vi "prueba5_21241028_ElminMejia.vi"() -> ()   [LabVIEW 2012]
panel:
  out "Array":T1(array[cluster]) {"tanque3" scale=0.0..10.0; "tanque2" scale=0.0..10.0; "tanque1" scale=0.0..10.0}
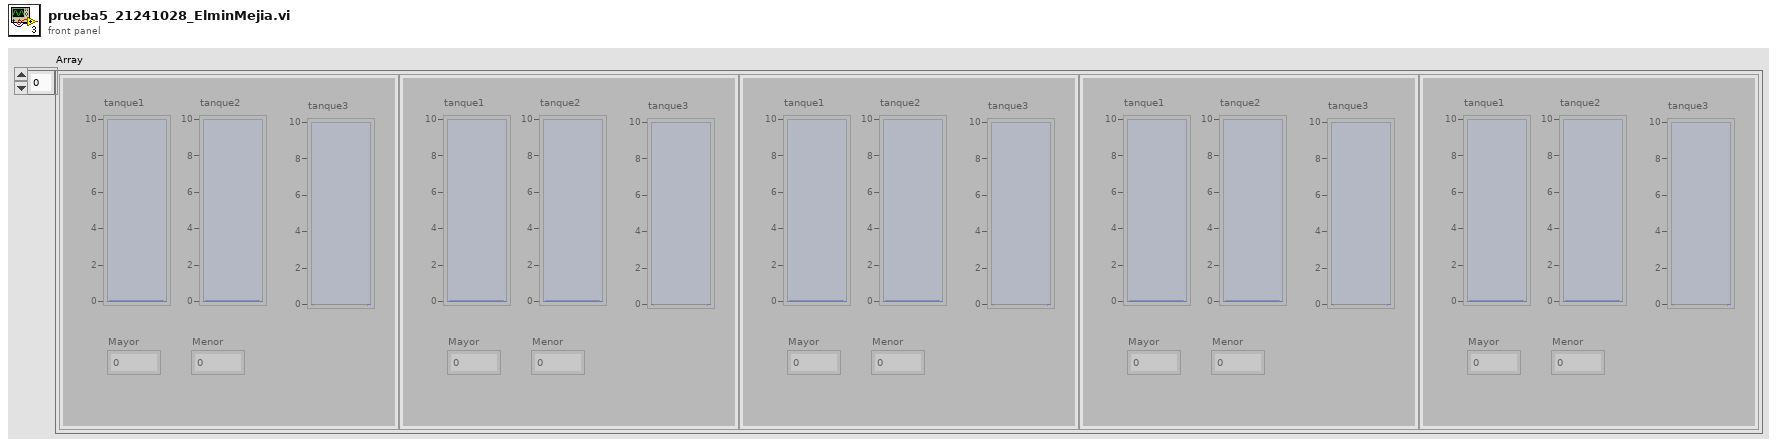
[diagram p1: front panel]
types:
  T1 = cluster{"tanque1":i32, "tanque2":i32, "tanque3":i32, "Mayor":dbl, "Menor":dbl}[]
  T2 = enum16{"open", "replace", "create", "open or create", "replace or create", "replace or create with confirmation"}
  T3 = cluster{"tanque1":i32, "tanque2":i32, "tanque3":i32, "Mayor":dbl, "Menor":dbl}
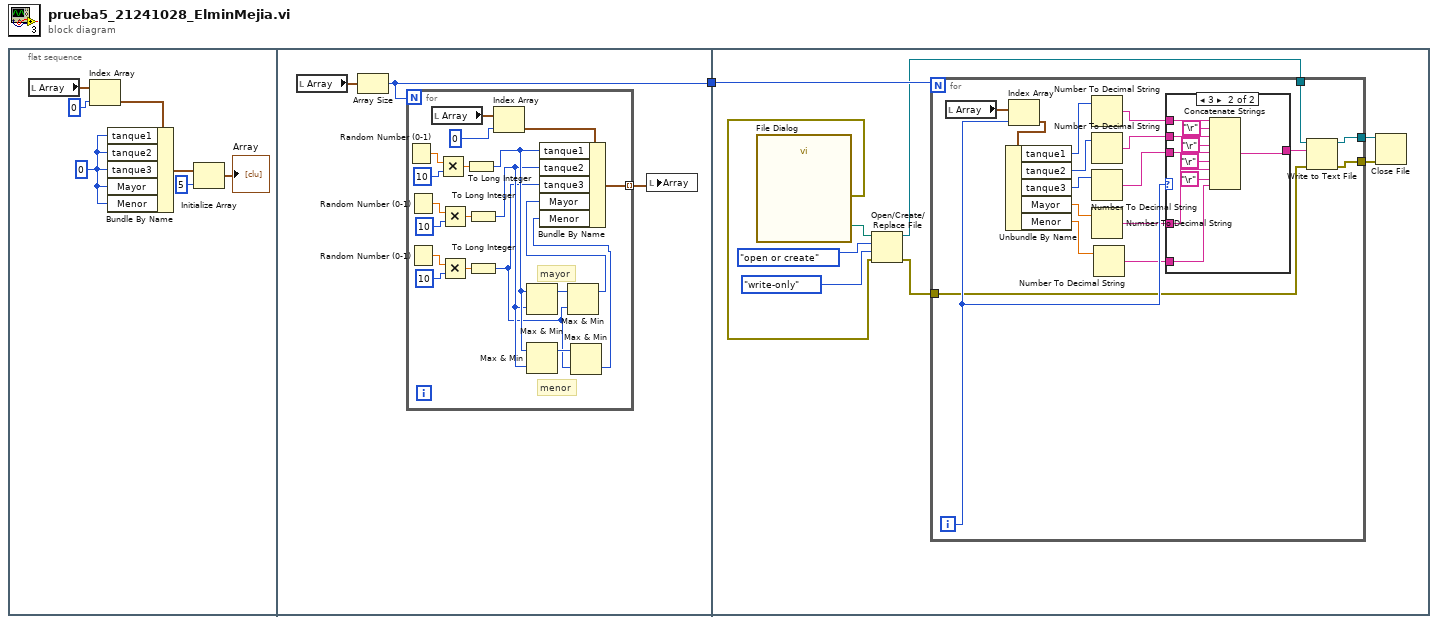
[diagram p0: block diagram]
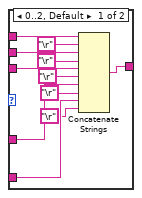
[diagram p2: hidden frame]
diagram:
  n1 = flat-sequence {
    tunnel: [w9] -> w1
    tunnel: w1 -> [w40]
    frame #0 {
      w5 = 0
      n2 = local read "Array"() -> (w8:T1)
      n3 = Index Array(array=w8, index=0) -> (element=w6:T3)
      n4 = Bundle By Name(cluster=w6, "tanque1"=w5, "tanque2"=w5, "tanque3"=w5, "Mayor"=w5, "Menor"=w5) -> (w4:T3)
      n5 = Initialize Array(w4, 5 ("dimension size")) -> (→"Array":T1)
    }
    frame #1 {
      n6 = local read "Array"() -> (w11:T1)
      n7 = Array Size(array=w11) -> (size(s)=w9:i32)
      n8 = for {
        N: w9 -> [_]
        tunnel: [w12] -> w10 mode=indexing
        # "menor"
        # "mayor"
        n9 = Random Number (0-1)() -> (number: 0 to 1=w28:dbl)
        n10 = Random Number (0-1)() -> (number: 0 to 1=w23:dbl)
        n11 = Random Number (0-1)() -> (number: 0 to 1=w22:dbl)
        n12 = local read "Array"() -> (w31:T1)
        n13 = Multiply(x=w28, y=10) -> (x*y=w26:dbl)
        n14 = Multiply(x=w23, y=10) -> (x*y=w25:dbl)
        n15 = Multiply(x=w22, y=10) -> (x*y=w20:dbl)
        n16 = To Long Integer(number=w26) -> (32bit integer=w17:i32)
        n17 = To Long Integer(number=w25) -> (32bit integer=w16:i32)
        n18 = To Long Integer(number=w20) -> (32bit integer=w14:i32)
        n19 = Index Array(array=w31, index=0) -> (element=w29:T3)
        n20 = Max & Min(x=w17, y=w16) -> (max(x,y)=w19:i32)  [unwired: 1 out]
        n21 = Max & Min(x=w17, y=w16) -> (max(x,y)=w15:i32)  [unwired: 1 out]
        n22 = Max & Min(x=w19, y=w14) -> (max(x,y)=w18:i32)  [unwired: 1 out]
        n23 = Max & Min(x=w15, y=w14) -> (min(x,y)=w13:i32)  [unwired: 1 out]
        n24 = Bundle By Name(cluster=w29, "tanque1"=w17, "tanque2"=w16, "tanque3"=w14, "Mayor"=w18, "Menor"=w13) -> (w12:T3)
      }
      n25 = local write "Array"(w10) -> ()
    }
    frame #2 {
      n26 = call "File Dialog"() -> ("selected path"=w39:path, "error out"=w38:errorcluster)  [unwired: 12 in, 2 out]
      n27 = Open/Create/Replace File(file path (use dialog)=w39, error in=w38, operation (0:open)=T2."open or create", access (0:read/write)=enum16{"read/write", "read-only", "write-only"}."write-only") -> (refnum out=w35:refnum<file>, error out=w34:errorcluster)  [unwired: 2 in, 1 out]
      n28 = for {
        N: w40 -> [_]
        tunnel: w35 -> [w44]
        tunnel: w34 -> [w43]
        tunnel: [w42] -> w33
        tunnel: [w41] -> w32
        i -> [w51]
        n29 = local read "Array"() -> (w58:T1)
        n30 = Index Array(array=w58, index=w51) -> (element=w57:T3)
        n31 = Unbundle By Name(w57) -> ("tanque1"=w56:i32, "tanque2"=w55:i32, "tanque3"=w54:i32, "Mayor"=w53:dbl, "Menor"=w52:dbl)
        n32 = Number To Decimal String(number=w56) -> (decimal integer string=w50:string)  [unwired: 1 in]
        n33 = Number To Decimal String(number=w55) -> (decimal integer string=w49:string)  [unwired: 1 in]
        n34 = Number To Decimal String(number=w54) -> (decimal integer string=w48:string)  [unwired: 1 in]
        n35 = Number To Decimal String(number=w53) -> (decimal integer string=w47:string)  [unwired: 1 in]
        n36 = Number To Decimal String(number=w52) -> (decimal integer string=w46:string)  [unwired: 1 in]
        n37 = case shown="3" w51 {
          tunnel: w50 -> [w69 w79]
          tunnel: w49 -> [w68 w78]
          tunnel: w48 -> [w67 w77]
          tunnel: w47 -> [w66 w76]
          tunnel: w46 -> [w65 w75]
          tunnel: [w59 w70] -> w45
          frame 0..2, Default {
            n38 = Concatenate Strings(w69, "\r", w68, "\r", w67, "\r", w66, "\r", w65, "\r") -> (w59:string)
          }
          frame 3 {
            n39 = Concatenate Strings(w79, "\r", w78, "\r", w77, "\r", w76, "\r", w75) -> (w70:string)
          }
        }
        n40 = Write to Text File(file (use dialog)=w44, text=w45, error in=w43) -> (refnum out=w42:refnum<file>, error out=w41:errorcluster)  [unwired: 1 in, 1 out]
      }
      n41 = Close File(refnum=w33, error in=w32) -> ()  [unwired: 2 out]
    }
  }
